vi "PID_Discipline_WithoutSystem_X72_Single_delay.vi"(0 "SR620_No.1_Port":refnum<visa-resource-name>="GPIB0::20::INSTR", 1 "Channel (1: A)":i32(ring)=1 items=["Ext Input", "A", "B"], 2 "SR620_No.1 (1: REF)":i32(ring) items=["A", "B", "REF", "A / B"], 3 "Meas. Mode (0: Time)":i32(ring) items=["Time", "Width", "Rise / Fall Time", "Frequency", "Period", "Phase", "Count"], 4 "Arming Mode (0: +/-time)":i32(ring)=1 items=["+/-time", "+time", "1 period", "0.01s gate", "0.1s gate", "1.0s gate", "ext trig +/- time", "ext trig +time", "ext gate/+ time/hldf", "ext triggered 1 period", "ext triggered .01s gate", "ext triggered 0.1s gate", "ext triggered 1.0s gate"], 5 "Gate Time (Auto)":dbl(ring) items=["Auto"=0.0, "1E-6"=1e-06, "2E-6"=2e-06, "5E-6"=5e-06, "1E-5"=1e-05, "2E-5"=2e-05, "5E-5"=5e-05, "1E-4"=0.0001, "2E-4"=0.0002, "5E-4"=0.0005, "1E-3"=0.001, "2E-3"=0.002, "5E-3"=0.005, ".01"=0.01, ".02"=0.02, ".05"=0.05, ".1"=0.1, ".2"=0.2, ".5"=0.5, "1"=1.0, "2"=2.0, "5"=5.0, "10"=10.0, "20"=20.0, "50"=50.0, "100"=100.0, "200"=200.0, "500"=500.0], 6 "Sample Size (1)":u32(ring)=1 items=["1"=1, "2"=2, "5"=5, "10"=10, "20"=20, "50"=50, "100"=100, "200"=200, "500"=500, "1000"=1000, "2000"=2000, "5000"=5000, "10000"=10000, "20000"=20000, "50000"=50000, "100000"=100000, "200000"=200000, "500000"=500000, "1000000"=1000000], 7 "SR620_No.1_error in (no error)1":errorcluster, 8 "Input Termination_ (0: 50 Ohms)":i32(ring) items=["50 Ohms", "1 Mohm", "UHF Prescalers"], 9 "Timeout (25000 ms)":u32=1000 step=1000, 10 "Coupling (F: DC)":bool, 11 "Ref Out (1: TTL)":i32(ring)=1 items=["ECL", "TTL"], 12 "Auto Trigger Level (True)":bool, 14 "Trigger Level (0.00 V)":dbl=1.0, 16 "Trigger Slope (T: Positive)":bool=TRUE) -> (20 "SR620_No.1":refnum<visa-resource-name>="GPIB0::20::INSTR", 27 "SR620_No1 error out":errorcluster)   [LabVIEW 2014]
doc: "Provides an example of how to use the SR620 subVIs programmatically."
uses:
  <vilib>/addons/control/pid/pid.llb/PID (DBL).vi
  <vilib>/Utility/file.llb/Write To Spreadsheet File (DBL).vi
  <vilib>/Instr/_visa.llb/VISA Configure Serial Port (Instr).vi
  <vilib>/addons/control/pid/NI_PID_pid.lvlib
panel:
  in  "是否延时":bool
  out "一次循环所需时间":u32
  out "本地测量钟差":dbl[](graph)=[7593300.0, 241.375901, 241.375903, 241.375876, 241.375868, 241.375803, 241.375857, 241.375887, 241.375852, 241.37583800000002, 241.37586299999998]
  in  "开始绘图":bool
  in  "delimiter (\\n)":string="\n" caption="数据分隔符(\\n)"
  in  "文件路径: single":path=path "C:/Users/Administrator/Desktop/PID_Discipline_WithoutSystem_X72_Single/single_read_data.txt"
  out "是否清零":dbl
  out "钟差改变量":dbl format="%#_10g"
  in  "驯服阈值(ns)":dbl=100.0
  out "驯服":bool
  out "当前粗调调整量（100ns）":i64
  in  "FPGA串口地址":refnum<visa-resource-name>="COM6"
  out "串口读取数值":i64
  out "读取缓冲区 （16进制）":string
  out "写入字符串2":string
  out "写入字符串1":string="0"
  out "最终粗调调整量（100ns）":i64
  in  "output range":cluster{"output high":dbl, "output low":dbl}={"output high"=400.0, "output low"=-400.0} caption="输出范围" {"output low" format="%.2f"; "output high" format="%.2f"}
  in  "PID gains":T1={"proportional gain (Kc)"=0.5, "integral time (Ti, min)"=0.0, "derivative time (Td, min)"=0.0} caption="PID增益" {"derivative time (Td, min)" format="%.3f"; "integral time (Ti, min)" format="%.3f"; "proportional gain (Kc)" format="%.3f"}
  out "反馈值":dbl format="%#.6f"
  in  "setpoint":dbl caption="设定值" format="%.3f"
  out "dt out (s)":dbl=1.0000000474974513 caption="dt输出(s)" format="%.3f"
  out "output":dbl caption="PID输出" format="%#.6f"
  in  "baud rate (9600) 2":u32=57600 caption="波特率(9600)"
  in  "VISA resource name 2":refnum<visa-resource-name>="COM3" caption="VISA资源名称"
  out "错误输出 2":errorcluster caption="错误输出"
  in  "baud rate (9600) 1":u32=57600 caption="波特率(9600)"
  in  "VISA resource name 1":refnum<visa-resource-name>="COM3" caption="VISA资源名称"
  out "错误输出 1":errorcluster caption="错误输出"
  out "串口工作":bool
  out "命令":string
  out "SR620_Delta_T":dbl format="%.12f"
  in  "等待时间（ms)":u32=1000
  out "总计数值":i32
  # "串口"
  # "数据处理"
  # "钟差调整量（ns）"
  # "数据显示及波形显示区域"
  # "公共调节区域"
  # "分别设置区域"
  # "Delta_T"
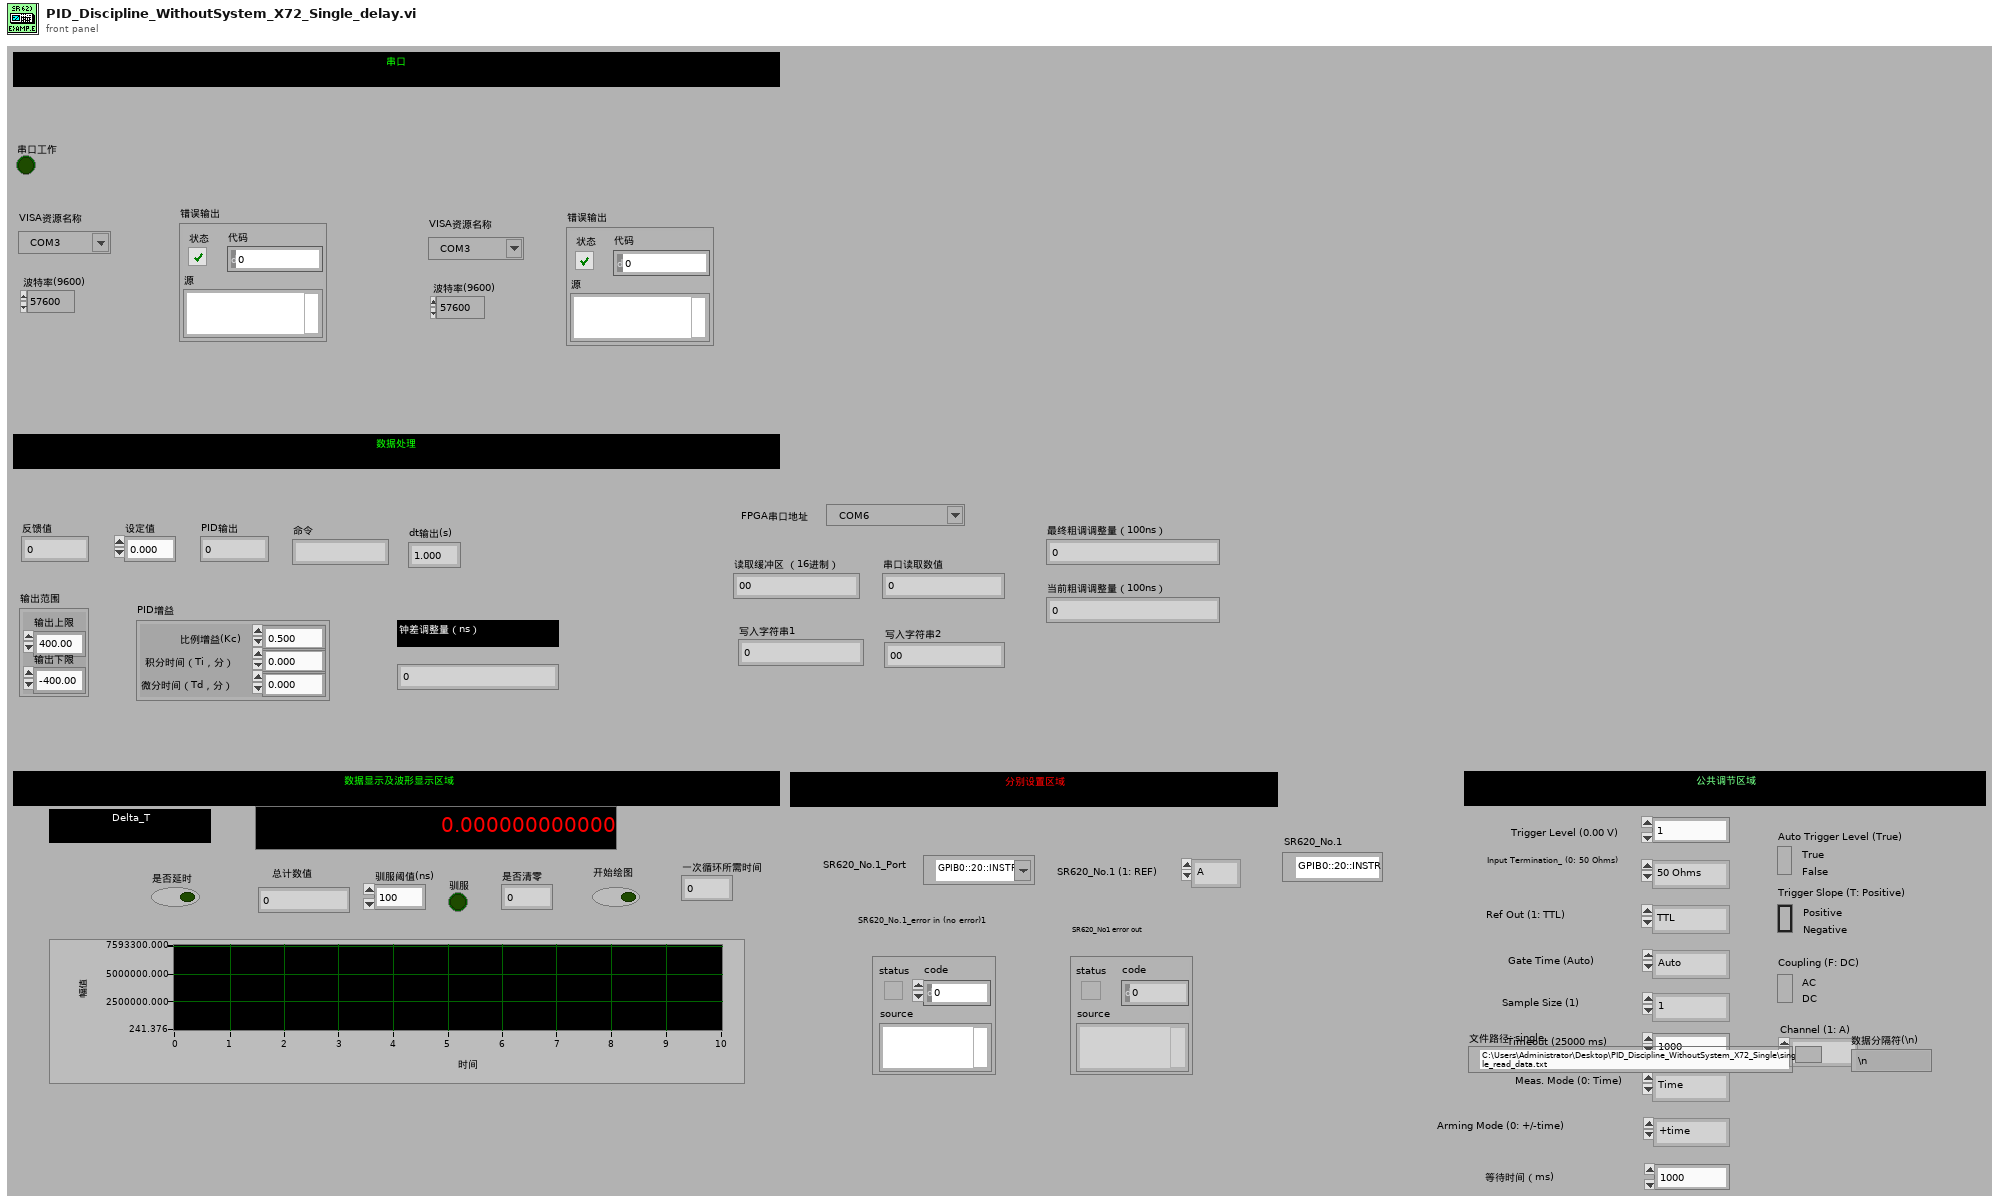
[diagram p1: front panel]
types:
  T1 = cluster{"proportional gain (Kc)":dbl, "integral time (Ti, min)":dbl, "derivative time (Td, min)":dbl}
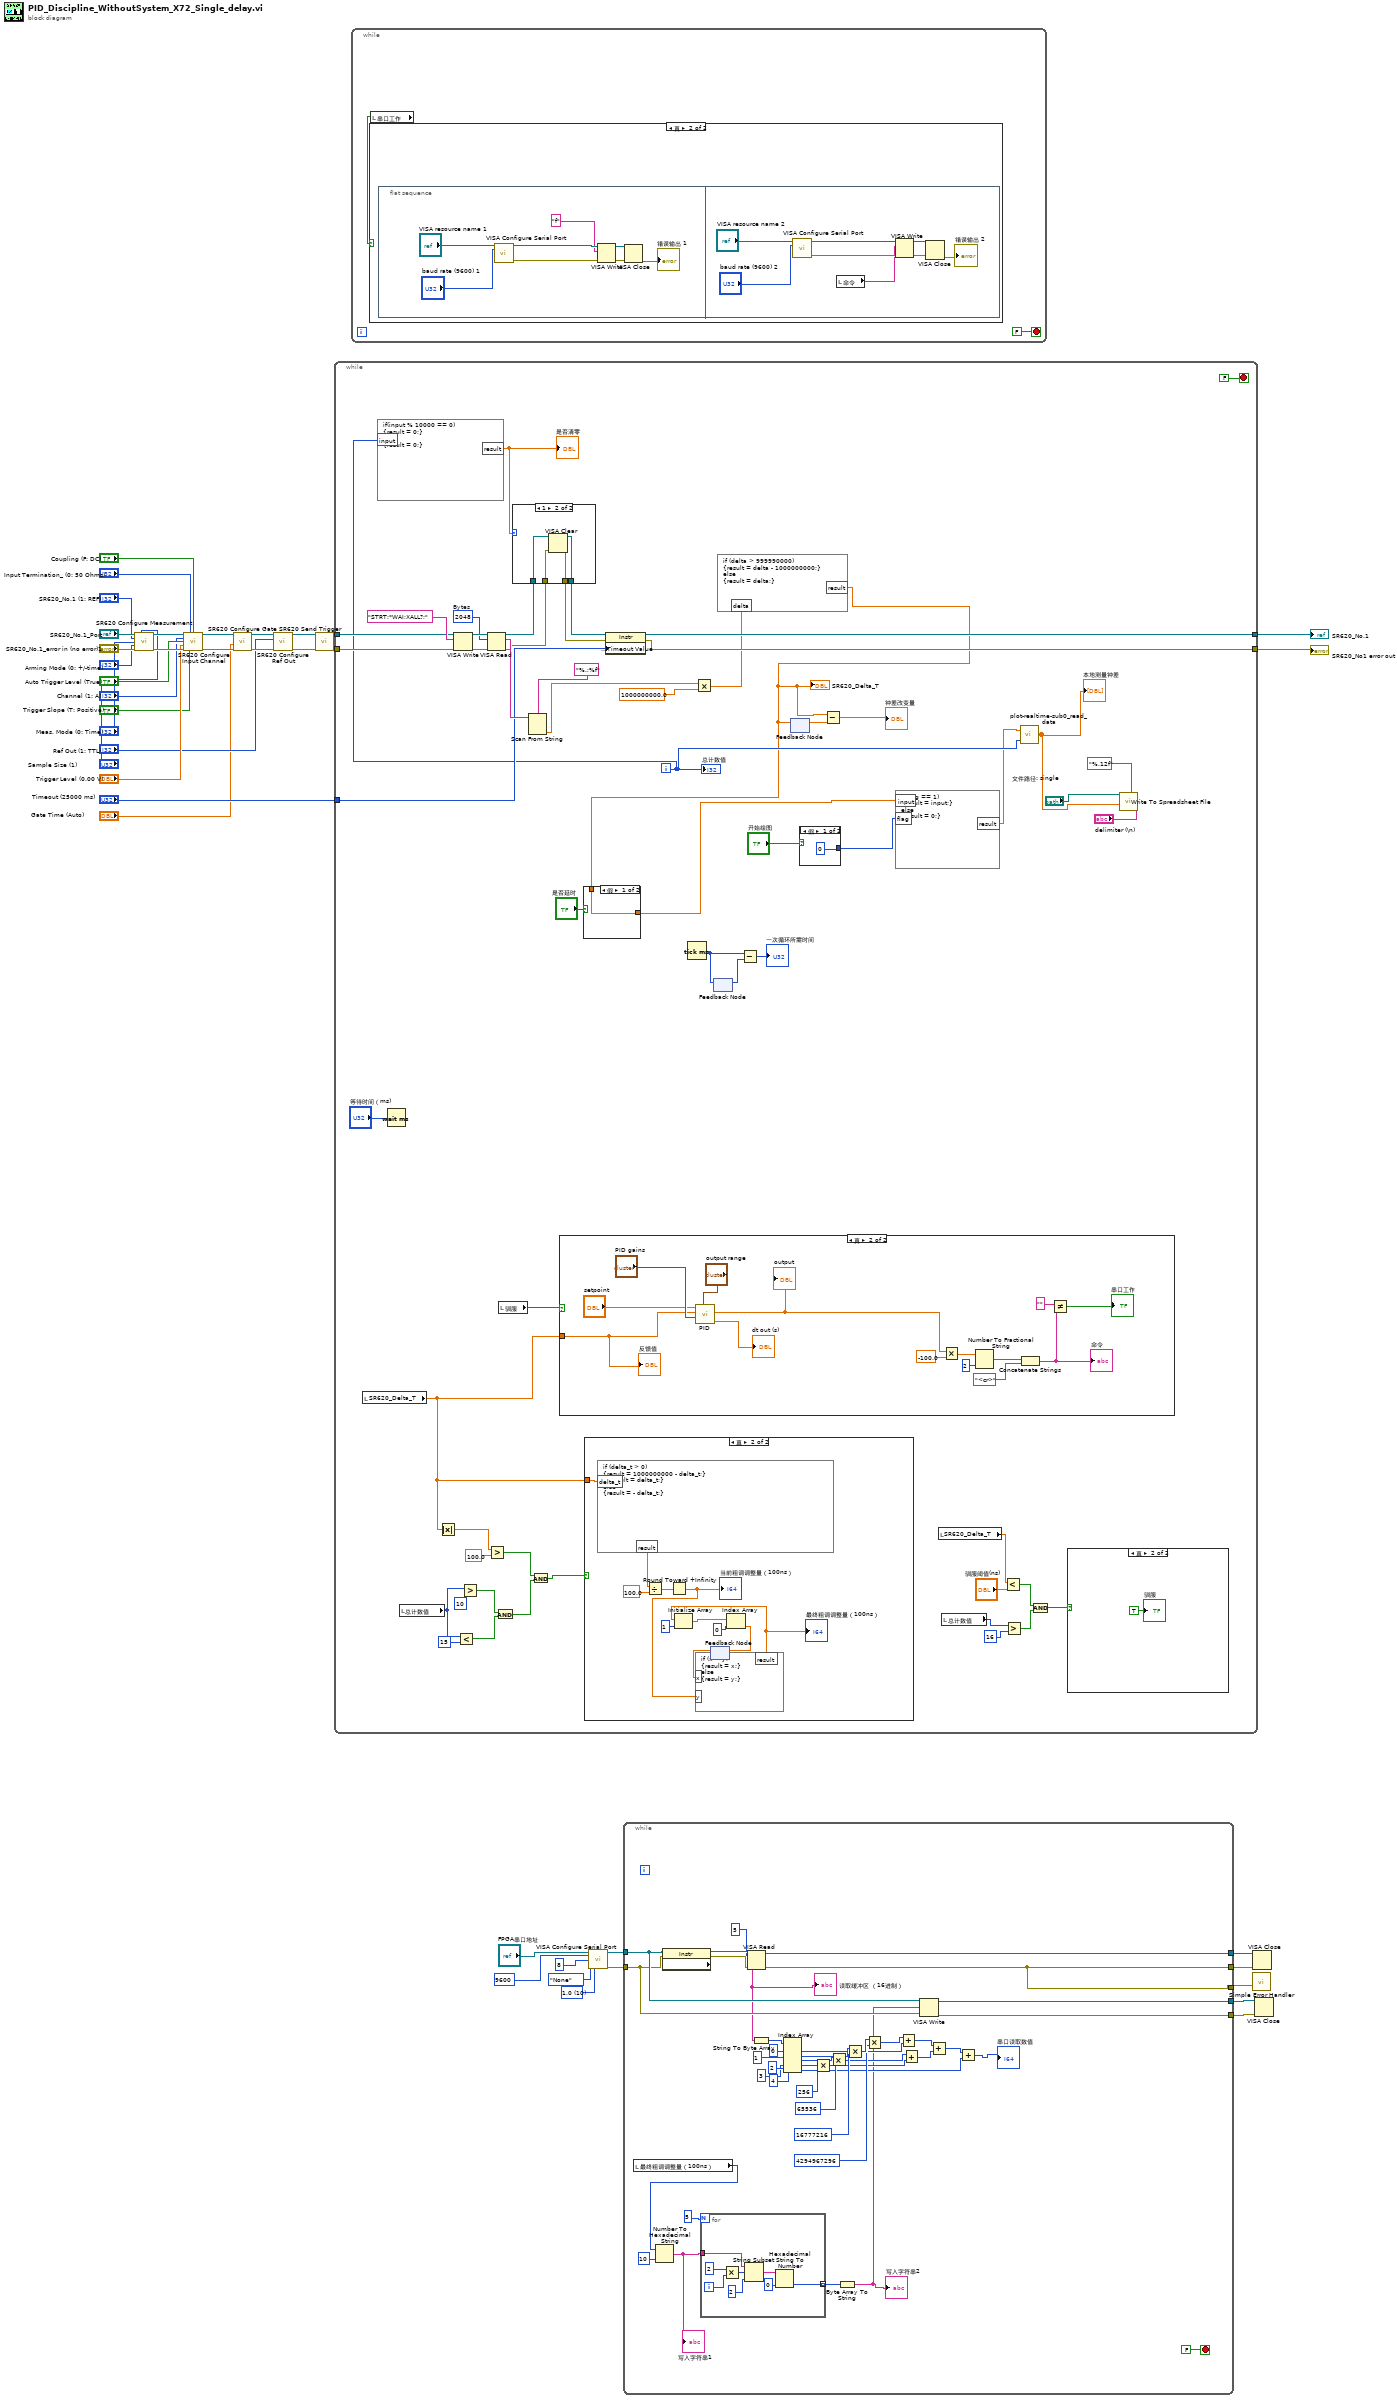
[diagram p0: block diagram]
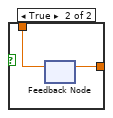
[diagram p3: hidden frame]
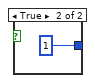
[diagram p4: hidden frame]
diagram:
  w20 = u16 10 items=["1.0"=10, "1.5"=15, "2.0"=20] ("stop bits (10: 1 bit)")
  n1 = call "SR620 Configure Measurement.vi"("VISA session"="SR620_No.1_Port", "Sample Size (1)"="Sample Size (1)", "Source (2: REF)"="SR620_No.1 (1: REF)", "Measurement Mode (0: Time)"="Meas. Mode (0: Time)", "Arming Mode (0: +/-time)"="Arming Mode (0: +/-time)", "error in (no error)"="SR620_No.1_error in (no error)1") -> ("dup VISA session"=w30:refnum<visa-resource-name>, "error out"=w28:errorcluster)  [unwired: 8 in]
  n2 = call "SR620 Configure Input Channel.vi"("VISA session"=w30, "Input Termination (0: 50 Ohms)"="Input Termination_ (0: 50 Ohms)", "Coupling (F: DC)"="Coupling (F: DC)", "Channel (1: A)"="Channel (1: A)", "Auto Trigger Level (True)"="Auto Trigger Level (True)", "Trigger Level (0.00 V)"="Trigger Level (0.00 V)", "error in (no error)"=w28, "Trigger Slope (T: Positive)"="Trigger Slope (T: Positive)") -> ("dup VISA session"=w29:refnum<visa-resource-name>, "error out"=w27:errorcluster)  [unwired: 6 in]
  n3 = call "SR620 Configure Gate.vi"("error in (no error)"=w27, "Gate Time (Auto)"="Gate Time (Auto)", "VISA session"=w29) -> ("error out"=w32:errorcluster, "dup VISA session"=w31:refnum<visa-resource-name>)  [unwired: 5 in]
  n4 = call "SR620 Configure Ref Out.vi"("error in (no error)"=w32, "Amplitude: Ref Output (1: TTL)"="Ref Out (1: TTL)", "VISA session"=w31) -> ("error out"=w33:errorcluster, "dup VISA session"=w34:refnum<visa-resource-name>)  [unwired: 3 in]
  n5 = call "SR620 Send Trigger.vi"("VISA session"=w34, "error in (no error)"=w33) -> ("dup VISA session"=w38:refnum<visa-resource-name>, "error out"=w37:errorcluster)  [unwired: 12 in]
  n6 = while "While循环" {
    tunnel: w38 -> [w89]
    tunnel: w37 -> [w88]
    tunnel: "Timeout (25000 ms)" -> [w65]
    tunnel: [w87] -> w25
    tunnel: [w86] -> w24
    i -> [w53]
    stop <- FALSE stop-if-true
    w93 = u32 2048  # Bytes
    n7 = local read "SR620_Delta_T"() -> (w60:dbl)
    n8 = formula code="if(input % 10000 == 0)\n{result = 0;}\nelse\n{result = 0;}"("input"=w53) -> ("result"=w54:dbl)
    "是否清零" <- w54
    n9 = Wait (ms)(milliseconds to wait="等待时间（ms)") -> ()  [unwired: 1 out]
    n10 = local read "总计数值"() -> (w80:i32)
    n11 = Absolute Value(x=w60) -> (abs(x)=w66:dbl)
    n12 = VISA Write(VISA resource name=w89, write buffer="STRT;*WAI;XALL?;" ("write buffer (\"\")"), error in (no error)=w88) -> (VISA resource name out=w94:refnum<visa-resource-name>, error out=w95:errorcluster)  [unwired: 1 out]
    n13 = Less?(x=w80, y=15) -> (x < y?=w77:bool)
    n14 = Greater?(x=w80, y=10) -> (0:w78:bool)
    n15 = VISA Read(VISA resource name=w94, byte count=w93, error in (no error)=w95) -> (VISA resource name out=w59:refnum<visa-resource-name>, read buffer=w90:string, error out=w57:errorcluster)  [unwired: 1 out]
    n16 = Greater?(x=w66, y=100.0) -> (0:w76:bool)
    n17 = And(x=w78, y=w77) -> (x .and. y?=w75:bool)
    n18 = local read "驯服"() -> (w68:bool)
    n19 = case shown="1" w54 {
      tunnel: w59 -> [w102 w106]
      tunnel: [w102 w105] -> w58
      tunnel: w57 -> [w101 w104]
      tunnel: [w101 w103] -> w56
      frame 0, Default {
      }
      frame 1 {
        n20 = VISA Clear(VISA resource name=w106, error in (no error)=w104) -> (VISA resource name out=w105:refnum<visa-resource-name>, error out=w103:errorcluster)
      }
    }
    n21 = Scan From String(format string="%.;%f", input string=w90) -> (output 1=w84:dbl)  [unwired: 3 in, 3 out]
    n22 = And(x=w76, y=w75) -> (x .and. y?=w74:bool)
    n23 = case shown="真" w68 {
      tunnel: w60 -> [_ w128]
      frame False {
      }
      frame True {
        n24 = call-poly <vilib>:"PID.vi"("output range"="output range", "PID gains"="PID gains", "process variable"=w128, "setpoint"="setpoint") -> ("dt out (s)"=→"dt out (s)":dbl, "output"=w120:dbl)  [unwired: 6 in]
        "output" <- w120
        n25 = Multiply(x=w120, y=-100.0) -> (x*y=w119:dbl)
        n26 = Number To Fractional String(number=w119, precision (6)=i16 2 ("精度(6)")) -> (F-format string=w126:string)  [unwired: 2 in]
        n27 = Concatenate Strings(w126, "<cr>" ("字符串")) -> (w122:string)
        "命令" <- w122
        n28 = Not Equal?(x="", y=w122) -> (x != y?=→"串口工作":bool)
        "反馈值" <- w128
      }
    }
    n29 = case shown="真" w74 {
      tunnel: w60 -> [_ w108]
      frame False {
      }
      frame True {
        n30 = formula code="if (delta_t > 0)\n{result = 1000000000 - delta_t;}\n//{result = delta_t;}\nelse\n{result = - delta_t;}"("delta_t"=w108) -> ("result"=w117:dbl)
        n31 = Divide(x=w117, y=100.0) -> (x/y=w116:dbl)
        n32 = Round Toward +Infinity(x=w116) -> (ceil(x): smallest int >= x=w110:dbl)
        "当前粗调调整量（100ns）" <- w110
        n33 = feedback #1() -> (w111:dbl)  [unwired: 1 in]
        n34 = formula code="if (x > y)\n{result = x;}\nelse\n{result = y;}"("x"=w111, "y"=w110) -> ("result"=w109:dbl)
        "最终粗调调整量（100ns）" <- w109
        n35 = Initialize Array(w109, 1 ("维数大小")) -> (w113:dbl[])
        n36 = Index Array(array=w113, index=0 ("索引")) -> (element=w112:dbl)
        n37 = feedback-in #1(w112) -> ()
      }
    }
    n38 = property class="Instr"(reference=w58, error in=w56, "General Settings:Timeout Value"=w65) -> (reference out=w87:refnum<visa-resource-name>, error out=w86:errorcluster)
    n39 = Tick Count (ms)() -> (millisecond timer value=w45:u32)
    n40 = Multiply(x=w84, y=1000000000.0) -> (x*y=w61:dbl)
    n41 = feedback #2() -> (w44:u32)  [unwired: 1 in]
    n42 = feedback-in #2(w45) -> ()
    n43 = formula code="if (delta > 999990000)\n{result = delta - 1000000000;}\nelse\n{result = delta;}"("delta"=w61) -> ("result"=w41:dbl)
    "SR620_Delta_T" <- w41
    n44 = case shown="假" "是否延时" {
      tunnel: w41 -> [w96 w98]
      tunnel: [w96 w97] -> w40
      frame False {
      }
      frame True {
        n45 = feedback-in #3(w98) -> ()
        n46 = feedback #3() -> (w97:dbl)  [unwired: 1 in]
      }
    }
    n47 = Subtract(x=w45, y=w44) -> (x-y=→"一次循环所需时间":u32)
    n48 = feedback #4() -> (w64:dbl)  [unwired: 1 in]
    n49 = feedback-in #4(w41) -> ()
    n50 = case shown="假" "开始绘图" {
      tunnel: [0 1] -> w48
      frame False {
      }
      frame True {
      }
    }
    n51 = Subtract(x=w41, y=w64) -> (x-y=→"钟差改变量":dbl)
    n52 = formula code="if(flag == 1)\n{result = input;}\nelse\n{result = 0;}"("flag"=w48, "input"=w40) -> ("result"=w47:dbl)
    n53 = local read "SR620_Delta_T"() -> (w62:dbl)
    n54 = local read "总计数值"() -> (w73:i32)
    n55 = Less?(x=w62, y="驯服阈值(ns)") -> (x < y?=w71:bool)
    n56 = Greater?(x=w73, y=16) -> (0:w70:bool)
    n57 = call "plot-realtime-sub0_read_data.vi"("索引"=w53, "x"=w47) -> ("数组"=w46:dbl[])
    "本地测量钟差" <- w46
    n58 = And(x=w71, y=w70) -> (x .and. y?=w69:bool)
    n59 = case shown="真" w69 {
      frame False {
      }
      frame True {
        "驯服" <- TRUE
      }
    }
    n60 = call-poly <vilib>:"Write To Spreadsheet File.vi"("delimiter (\\t)"="delimiter (\\n)", "format (%.3f)"="%.12f", "1D data"=w46, "file path (dialog if empty)"="文件路径: single") -> ()  [unwired: 4 in, 1 out]
    "总计数值" <- w53
  }
  "SR620_No.1" <- w25
  "SR620_No1 error out" <- w24
  n61 = while {
    stop <- FALSE stop-if-true
    n62 = local read "串口工作"() -> (w133:bool)
    n63 = case shown="真" w133 {
      frame False {
      }
      frame True {
        n64 = flat-sequence {
          frame #0 {
            n65 = call-poly "VISA Configure Serial Port"("VISA resource name"="VISA resource name 1", "baud rate (9600)"="baud rate (9600) 1") -> ("VISA resource name out"=w142:refnum<visa-resource-name>, "error out"=w139:errorcluster)  [unwired: 12 in]
            n66 = VISA Write(VISA resource name=w142, write buffer="f" ("写入缓冲区"), error in (no error)=w139) -> (VISA resource name out=w137:refnum<visa-resource-name>, error out=w136:errorcluster)  [unwired: 1 out]
            n67 = VISA Close(VISA resource name=w137, error in (no error)=w136) -> (error out=→"错误输出 1":errorcluster)
          }
          frame #1 {
            n68 = call-poly "VISA Configure Serial Port"("VISA resource name"="VISA resource name 2", "baud rate (9600)"="baud rate (9600) 2") -> ("VISA resource name out"=w147:refnum<visa-resource-name>, "error out"=w149:errorcluster)  [unwired: 12 in]
            n69 = local read "命令"() -> (w146:string)
            n70 = VISA Write(VISA resource name=w147, write buffer=w146, error in (no error)=w149) -> (VISA resource name out=w145:refnum<visa-resource-name>, error out=w144:errorcluster)  [unwired: 1 out]
            n71 = VISA Close(VISA resource name=w145, error in (no error)=w144) -> (error out=→"错误输出 2":errorcluster)
          }
        }
      }
    }
  }
  n72 = call-poly "VISA Configure Serial Port"("VISA resource name"="FPGA串口地址", "baud rate (9600)"=u32 9600, "data bits (8)"=u16 8, "parity (0:none)"=enum16{"None", "Odd", "Even", "Mark", "Space"}."None", "stop bits (10: 1 bit)"=w20) -> ("VISA resource name out"=w18:refnum<visa-resource-name>, "error out"=w17:errorcluster)  [unwired: 9 in]
  n73 = while {
    tunnel: w18 -> [w188]
    tunnel: w17 -> [w187]
    tunnel: [w185] -> w16
    tunnel: [w184] -> w15
    tunnel: [w184] -> w14
    tunnel: [w183] -> w13
    tunnel: [w182] -> w12
    stop <- FALSE stop-if-true
    n74 = local read "最终粗调调整量（100ns）"() -> (w152:i64)
    n75 = Number To Hexadecimal String(1:i16 10 ("宽度(-)"), 2:w152) -> (0:w154:string)
    "写入字符串1" <- w154
    n76 = property class="Instr" props=["Serial Settings:Number of Bytes at Serial Port"](reference=w188, error in=w187) -> (reference out=w190:refnum<visa-resource-name>, error out=w189:errorcluster)  [unwired: 1 out]
    n77 = for {
      N: 5 -> [_]
      tunnel: w154 -> [w194]
      tunnel: [w191] -> w156 mode=indexing
      i -> [w198]
      n78 = Multiply(x=2, y=w198) -> (x*y=w196:i32)
      n79 = String Subset(string=w194, offset (0)=w196, length (rest)=2) -> (substring=w193:string)
      n80 = Hexadecimal String To Number(string=w193, default (0uL)=u8 0 ("默认(0 U32)")) -> (number=w191:u8)  [unwired: 1 in, 1 out]
    }
    n81 = VISA Read(VISA resource name=w190, byte count=5, error in (no error)=w189) -> (VISA resource name out=w185:refnum<visa-resource-name>, read buffer=w158:string, error out=w184:errorcluster)  [unwired: 1 out]
    "读取缓冲区 （16进制）" <- w158
    n82 = String To Byte Array(string=w158) -> (unsigned byte array=w181:u8[])
    n83 = Index Array ("索引数组")(array=w181, index #1=0 ("索引"), index #2=1 ("索引"), index #3=2 ("索引"), index #4=3 ("索引"), index #5=4 ("索引")) -> (element #1=w169:u8, element #2=w170:u8, element #3=w172:u8, element #4=w173:u8, element #5=w160:u8)
    n84 = Multiply ("乘")(x=w173, y=i64 256) -> (x*y=w164:i64)
    n85 = Multiply ("乘")(x=w172, y=i64 65536) -> (x*y=w165:i64)
    n86 = Byte Array To String(unsigned byte array=w156) -> (string=w153:string)
    "写入字符串2" <- w153
    n87 = Multiply ("乘")(x=w170, y=i64 16777216) -> (x*y=w166:i64)
    n88 = Multiply ("乘")(x=w169, y=i64 4294967296) -> (x*y=w167:i64)
    n89 = Add ("加")(x=w167, y=w166) -> (x+y=w163:i64)
    n90 = Add ("加")(x=w165, y=w164) -> (x+y=w162:i64)
    n91 = VISA Write(VISA resource name=w188, write buffer=w153, error in (no error)=w187) -> (VISA resource name out=w183:refnum<visa-resource-name>, error out=w182:errorcluster)  [unwired: 1 out]
    n92 = Add ("加")(x=w163, y=w162) -> (x+y=w161:i64)
    n93 = Add ("加")(x=w161, y=w160) -> (x+y=→"串口读取数值":i64)
  }
  n94 = call <vilib>:"Simple Error Handler.vi"("error in (no error)"=w14) -> ()  [unwired: 4 in, 5 out]
  n95 = VISA Close(VISA resource name=w16, error in (no error)=w15) -> ()  [unwired: 1 out]
  n96 = VISA Close(VISA resource name=w13, error in (no error)=w12) -> ()  [unwired: 1 out]
